vi "Find Entity by Type.vi"(7 "Entity Type":refnum<class "Entity.lvclass">, 8 "error in (no error)":errorcluster, 9 "Column Criteria":refnum<class "Type.lvclass">, 10 "Types":refnum<class "Type.lvclass">[](array[class]), 11 "Database in":refnum<class "Database Platform.lvclass">) -> (0 "error out":errorcluster, 2 "Entity":refnum<class "Entity.lvclass">, 3 "Database out":refnum<class "Database Platform.lvclass">)   [LabVIEW 2020, in "Conditu2.lvlib" / "Database Platform.lvclass"]
uses:
  Database Platform.lvclass
  Columns/Type/Type.lvclass
  Entity/Entity.lvclass
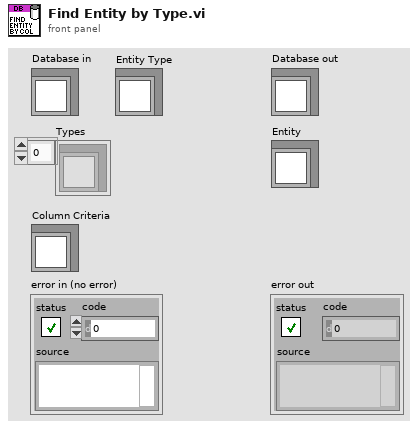
[diagram p1: front panel]
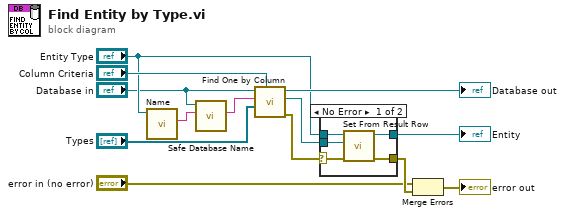
[diagram p0: block diagram]
diagram:
  n1 = call-dynamic "Name.vi"("Entity in"="Entity Type") -> ("Name"=w12:string)  [unwired: 10 in]
  n2 = call-dynamic "Safe Database Name.vi"("Conditum Name"=w12, "Database in"="Database in") -> ("Database Name"=w9:string)  [unwired: 9 in]
  n3 = call-dynamic "Find One by Column.vi"("Column Criteria"="Column Criteria", "Entity Definition"="Types", "Table Name"=w9, "Database in"="Database in") -> ("error out"=w7:errorcluster, "Result Row"=w8:refnum<class "Result Row.lvclass">, "Database out"=→"Database out":refnum<class "Database Platform.lvclass">)  [unwired: 5 in]
  n4 = case shown="No Error" w7 {
    selector: w7 -> [w16 w19]
    tunnel: "Entity Type" -> [w18 w20]
    tunnel: w8 -> [w17 _]
    tunnel: [w15 w20] -> w5
    tunnel: [w14 w19] -> w4
    frame No Error {
      n5 = call "Set From Result Row.vi"("error in (no error)"=w16, "Result Row"=w17, "Entity in"=w18) -> ("error out"=w14:errorcluster, "Entity out"=w15:refnum<class "Entity.lvclass">)  [unwired: 7 in]
    }
    frame Error {
    }
  }
  "Entity" <- w5
  n6 = Merge Errors("error in (no error)", w4) -> (→"error out":errorcluster)
